vi "Add Secondary Child.vi"(6 "Value":string, 8 "error in":errorcluster, 9 "Child":string, 10 "Parent":string, 11 "Tree Refnum in":refnum<vi>) -> (0 "error out":errorcluster, 3 "Tree Refnum out":refnum<vi>)   [LabVIEW 2019, in "Configuration.lvlib" / "Configuration.lvclass"]
uses:
  Configuration.lvclass
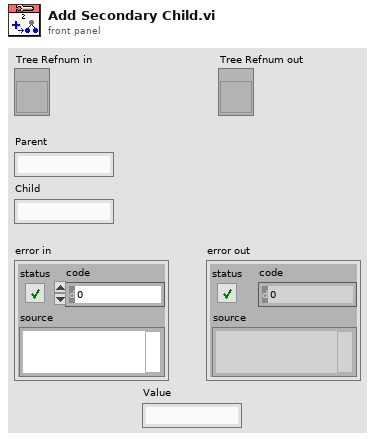
[diagram p1: front panel]
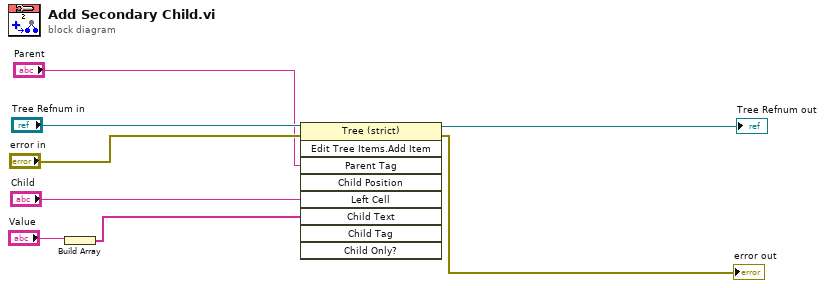
[diagram p0: block diagram]
diagram:
  n1 = Build Array("Value") -> (w1:string[])
  n2 = invoke class="Tree (strict)" method="Edit Tree Items.Add Item"(reference="Tree Refnum in", error in="error in", "Parent Tag"="Parent", "Left Cell"="Child", "Child Text"=w1) -> (reference out=→"Tree Refnum out":refnum<vi>, error out=→"error out":errorcluster)  [unwired: 4 in, 7 out]
